vi "LVCAM Initialize.vi"(10 "Self Actor":refnum<class "LVCAM.lvclass">, 11 "LVCAM Initialize in":refnum<class "LVCAM Initialize.lvclass">) -> (0 "error out":errorcluster, 3 "LVCAM Initialize out":refnum<class "LVCAM Initialize.lvclass">)   [LabVIEW 2021, in "LVCAM.lvlib" / "LVCAM Initialize.lvclass"]
uses:
  LVCAM Initialize.lvclass
  LVCAM/LVCAM.lvclass
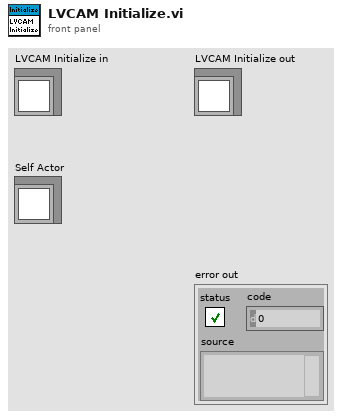
[diagram p1: front panel]
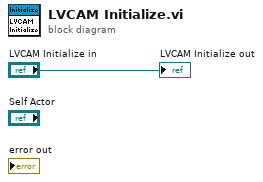
[diagram p0: block diagram]
diagram:
  "LVCAM Initialize out" <- "LVCAM Initialize in"
